vi "Find current file num.vi"() -> (0 "Current File Num":u16)   [LabVIEW 2013]
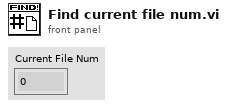
[diagram p1: front panel]
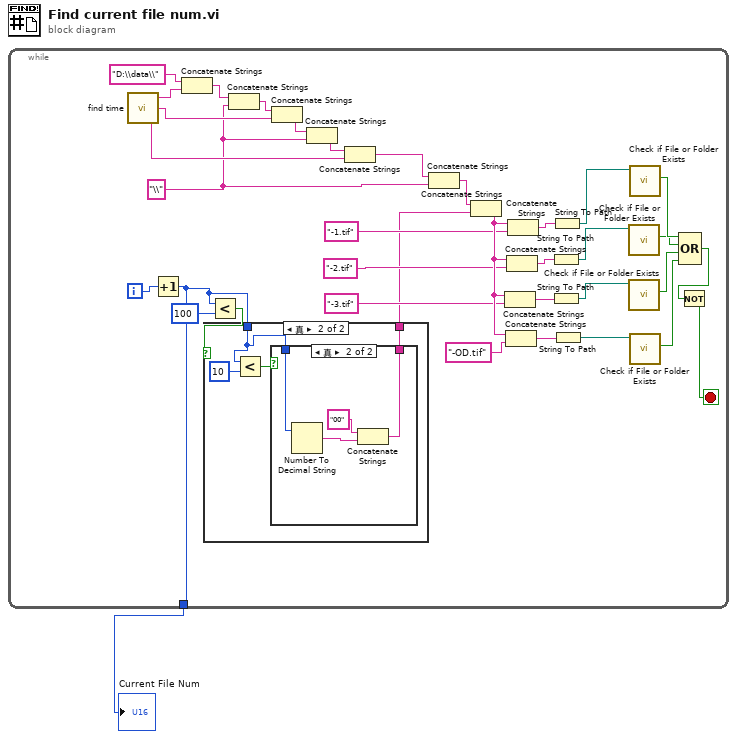
[diagram p0: block diagram]
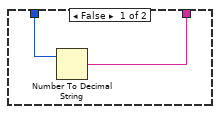
[diagram p2: hidden frame]
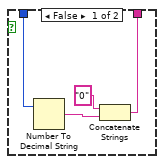
[diagram p3: hidden frame]
diagram:
  n1 = while {
    tunnel: [w3] -> w1
    i -> [w36]
    stop <- w6 stop-if-true
    w26 = "\\" ("字符串")
    n2 = call "find time.vi"() -> ("day"=w28:string, "month"=w31:string, "year"=w34:string)  [unwired: 3 in]
    n3 = Increment(x=w36) -> (x+1=w3:i32)
    n4 = Concatenate Strings("D:\\data\\", w34) -> (w33:string)
    n5 = Less?(x=w3, y=100) -> (x < y?=w4:bool)
    n6 = case shown="真" w4 {
      tunnel: w3 -> [w38 w40]
      tunnel: [w37 w39] -> w2
      frame False {
        n7 = Number To Decimal String(number=w38) -> (decimal integer string=w37:string)  [unwired: 1 in]
      }
      frame True {
        n8 = Less?(x=w40, y=10) -> (x < y?=w41:bool)
        n9 = case shown="真" w41 {
          tunnel: w40 -> [w44 w50]
          tunnel: [w43 w47] -> w39
          frame False {
            n10 = Number To Decimal String(number=w44) -> (decimal integer string=w46:string)  [unwired: 1 in]
            n11 = Concatenate Strings("0" ("字符串"), w46) -> (w43:string)
          }
          frame True {
            n12 = Number To Decimal String(number=w50) -> (decimal integer string=w49:string)  [unwired: 1 in]
            n13 = Concatenate Strings("00" ("字符串"), w49) -> (w47:string)
          }
        }
      }
    }
    n14 = Concatenate Strings(w33, w26) -> (w32:string)
    n15 = Concatenate Strings(w32, w31) -> (w30:string)
    n16 = Concatenate Strings(w30, w26) -> (w29:string)
    n17 = Concatenate Strings(w29, w28) -> (w27:string)
    n18 = Concatenate Strings(w27, w26) -> (w25:string)
    n19 = Concatenate Strings(w25, w2) -> (w23:string)
    n20 = Concatenate Strings(w23, "-3.tif" ("字符串")) -> (w16:string)
    n21 = Concatenate Strings(w23, "-OD.tif" ("字符串")) -> (w15:string)
    n22 = Concatenate Strings(w23, "-2.tif" ("字符串")) -> (w17:string)
    n23 = Concatenate Strings(w23, "-1.tif" ("字符串")) -> (w18:string)
    n24 = String To Path(string=w17) -> (path=w14:path)
    n25 = String To Path(string=w16) -> (path=w13:path)
    n26 = String To Path(string=w18) -> (path=w19:path)
    n27 = String To Path(string=w15) -> (path=w12:path)
    n28 = call <vilib>:"Check if File or Folder Exists.vi"("path"=w14) -> ("file or folder exists?"=w10:bool)  [unwired: 8 in, 2 out]
    n29 = call <vilib>:"Check if File or Folder Exists.vi"("path"=w13) -> ("file or folder exists?"=w9:bool)  [unwired: 8 in, 2 out]
    n30 = call <vilib>:"Check if File or Folder Exists.vi"("path"=w19) -> ("file or folder exists?"=w11:bool)  [unwired: 8 in, 2 out]
    n31 = call <vilib>:"Check if File or Folder Exists.vi"("path"=w12) -> ("file or folder exists?"=w8:bool)  [unwired: 8 in, 2 out]
    n32 = Compound Arithmetic op=OR(w11, w10, w9, w8) -> (w7:bool)
    n33 = Not(x=w7) -> (.not. x?=w6:bool)
  }
  "Current File Num" <- w1
